vi "Main.vi"() -> ()   [LabVIEW 2012]
uses:
  UIActionQueueElement.ctl
  UIAction.ctl
  MemoryGlobalAction.ctl
  ScanListGlobalAction.ctl
  TriggerConfigurationGlobalAction.ctl
  SlotConfigurationGlobalAction.ctl
  Setup.ctl
  SlotConfiguration.ctl
  BankConfiguration.ctl
  TriggerConfiguration.ctl
  TriggerArmConfiguration.ctl
  driver/Public/Controls/ArmSource.ctl
  TriggerScanConfiguration.ctl
  driver/Public/Controls/ScanSource.ctl
  TriggerChannelConfiguration.ctl
  driver/Public/Controls/TriggerSource.ctl
  HardwareActionQueueElement.ctl
  HardwareAction.ctl
  libs/LV-Utilities/LV-Utilities.lvlib
  driver/Keithley-7001.lvlib
panel:
  in  "Tab Control":enum32{"Page 1"}(tab)
  out "Setup File":path
  in  "CONFIGURE SLOT 1":bool
  in  "CONFIGURE MEMORY":bool
  in  "CONFIGURE SCAN":bool
  in  "CONFIGURE TRIGGER":bool
  in  "Hardware START":bool
  out "Hardware Running?":bool
  in  "RESET":bool
  in  "SAVE":bool
  in  "OPEN":bool
  in  "DONE":bool
  # "RUN"
  # "SETUP"
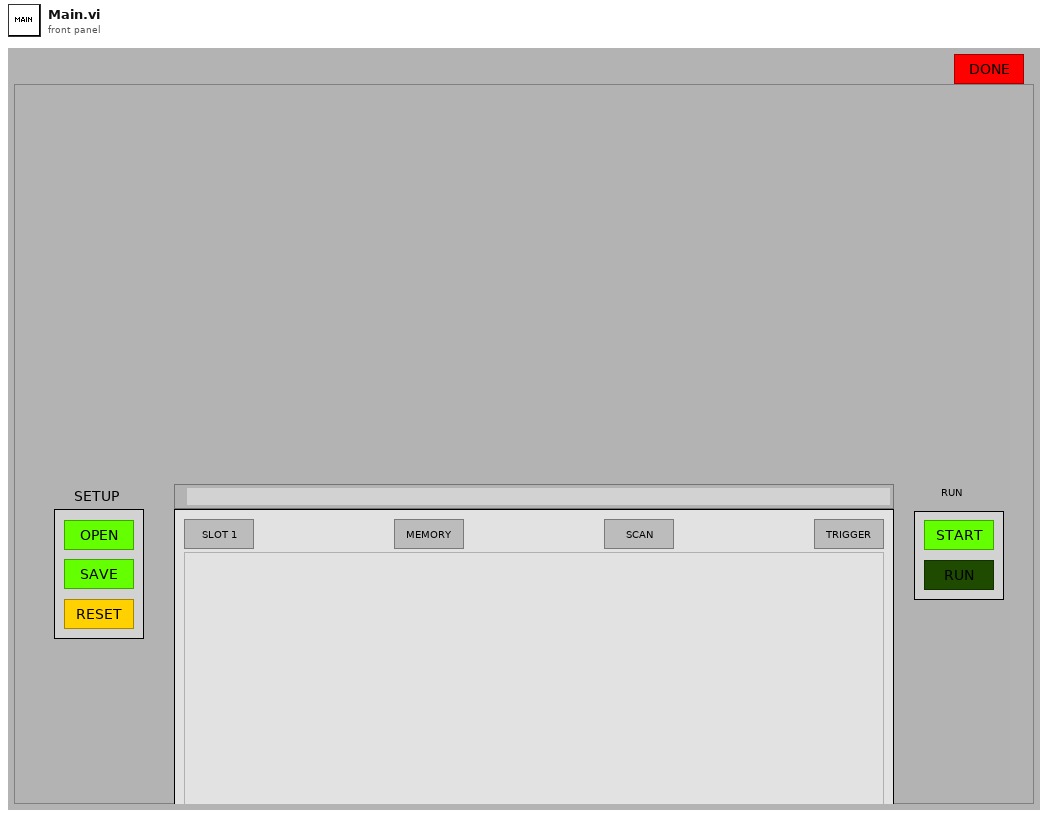
[diagram p1: front panel]
types:
  T1 = typedef "ActionQueues.ctl" = cluster{"User Interface":refnum<queue>, "Hardware":refnum<queue>}
  T2 = typedef "ExecutableConfiguration.ctl" = cluster{"GPIB ID":u8, "GPIB Board":u8, "Default Setup Folder":path}
  T3 = typedef "SlotConfigurationGlobalAction.ctl" = enum16{"Get", "Set", "Reset"}
  T4 = typedef "TriggerConfigurationGlobalAction.ctl" = enum16{"Get", "Set", "Reset"}
  T5 = typedef "ScanListGlobalAction.ctl" = enum16{"Get", "Set", "Reset"}
  T6 = typedef "MemoryGlobalAction.ctl" = enum16{"Get", "Set", "Reset"}
  T7 = typedef "Setup.ctl" = cluster{"Slots":T8[], "Memory":string[], "Scan List":string, "Trigger":T10}
  T8 = typedef "SlotConfiguration.ctl" = cluster{"Board":string, "Name":string, "Banks":T9[]}
  T9 = typedef "BankConfiguration.ctl" = cluster{"ID":string, "Name":string, "Channel Names":string[]}
  T10 = typedef "TriggerConfiguration.ctl" = cluster{"Arm":T11, "Scan":T13, "Channel":T15}
  T11 = typedef "TriggerArmConfiguration.ctl" = cluster{"Source":T12, "Count":u32, "Infinite?":bool}
  T12 = typedef "Keithley-7001.lvlib/ArmSource.ctl" = enum16{"Hold", "Immediate", "Manual", "Bus", "TLink", "External"}
  T13 = typedef "TriggerScanConfiguration.ctl" = cluster{"Source":T14, "Count":u32, "Infinite?":bool, "Delay (sec)":dbl, "Interval (sec)":dbl}
  T14 = typedef "Keithley-7001.lvlib/ScanSource.ctl" = enum16{"Hold", "Immediate", "Timer", "Manual", "Bus", "TLink", "External"}
  T15 = typedef "TriggerChannelConfiguration.ctl" = cluster{"Source":T16, "Count":u32, "Infinite?":bool, "Auto Count?":bool, "Delay (sec)":dbl, "Interval (sec)":dbl}
  T16 = typedef "Keithley-7001.lvlib/TriggerSource.ctl" = enum16{"Hold", "Immediate", "Manual", "Bus", "TLink", "External", "Timer"}
  T17 = typedef "HardwareActionQueueElement.ctl" = cluster{"Action":T18, "Data":variant}
  T18 = typedef "HardwareAction.ctl" = enum16{"Initialize", "Start", "Stop", "Error", "Shutdown"}
  T19 = typedef "UIActionQueueElement.ctl" = cluster{"Action":T20, "Data":variant}
  T20 = typedef "UIAction.ctl" = enum16{"Initialize", "Configure Trigger", "Configure Scan", "Configure Memory", "Configure Slot 1", "Open", "Save", "Reset", "Start", "Started", "Stop", "Stopped", "Shutdown"}
  T21 = enum8{"Enabled", "Disabled", "Disabled and Grayed Out"}
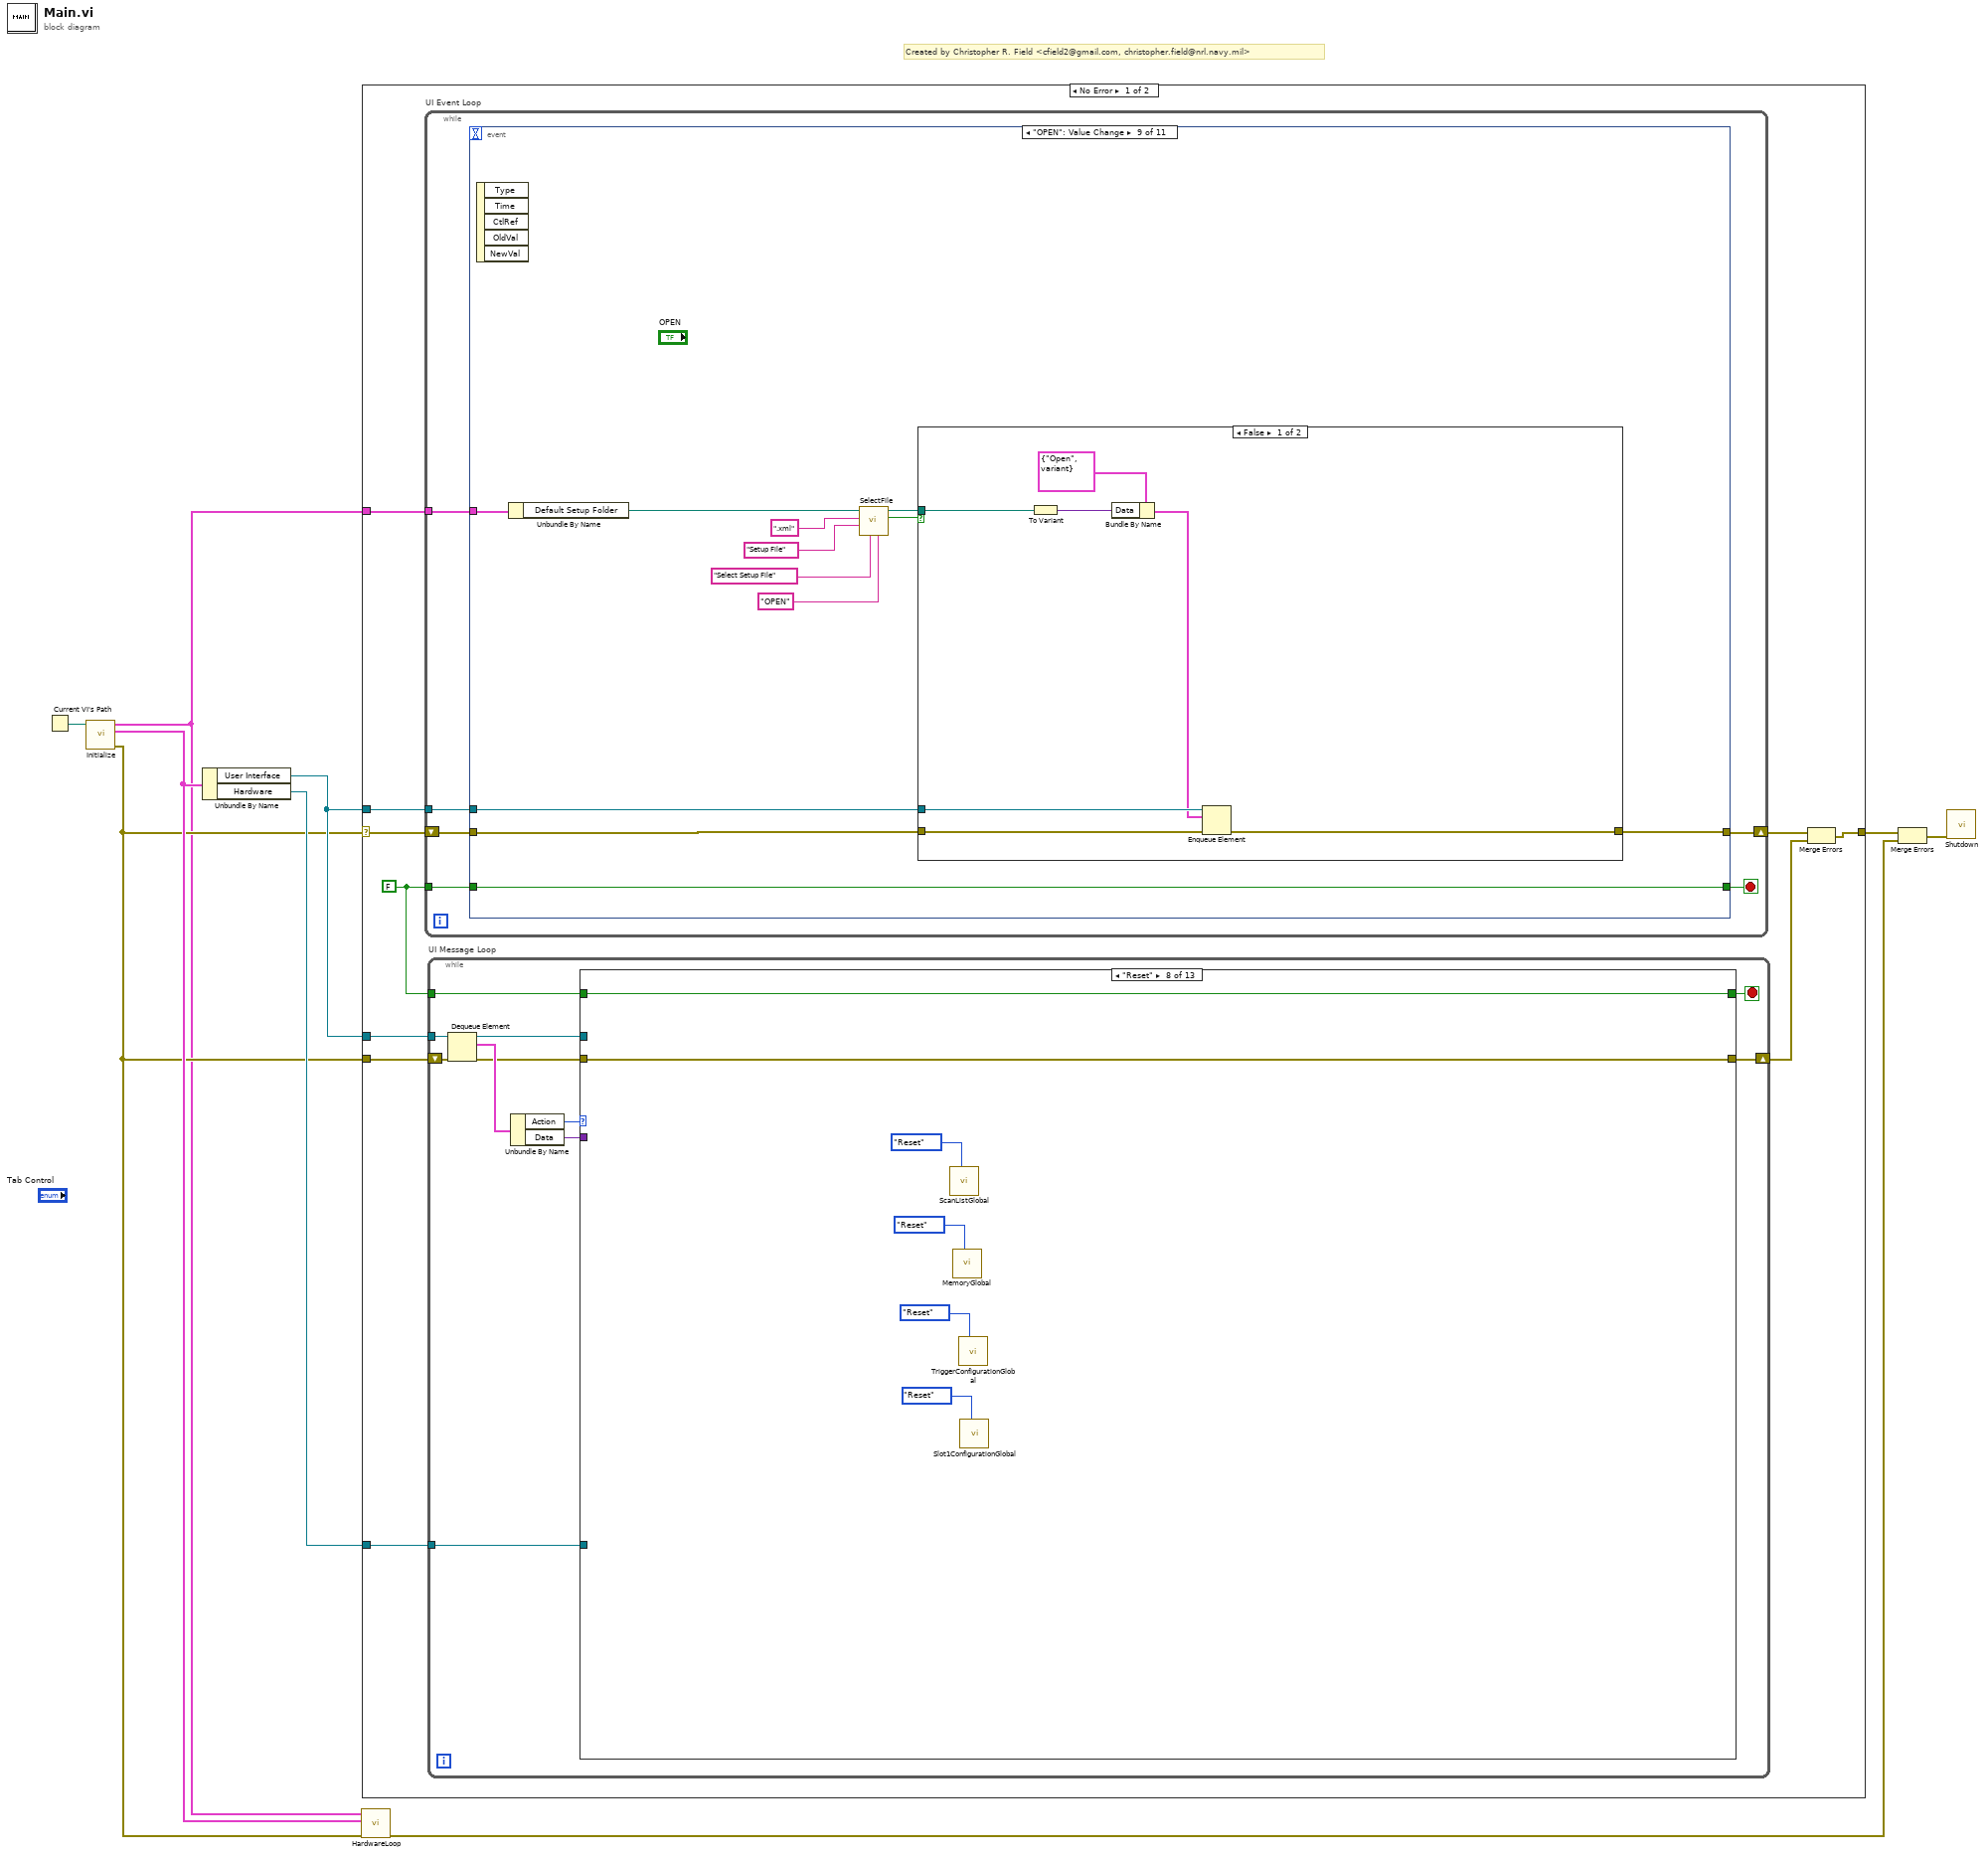
[diagram p0: block diagram]
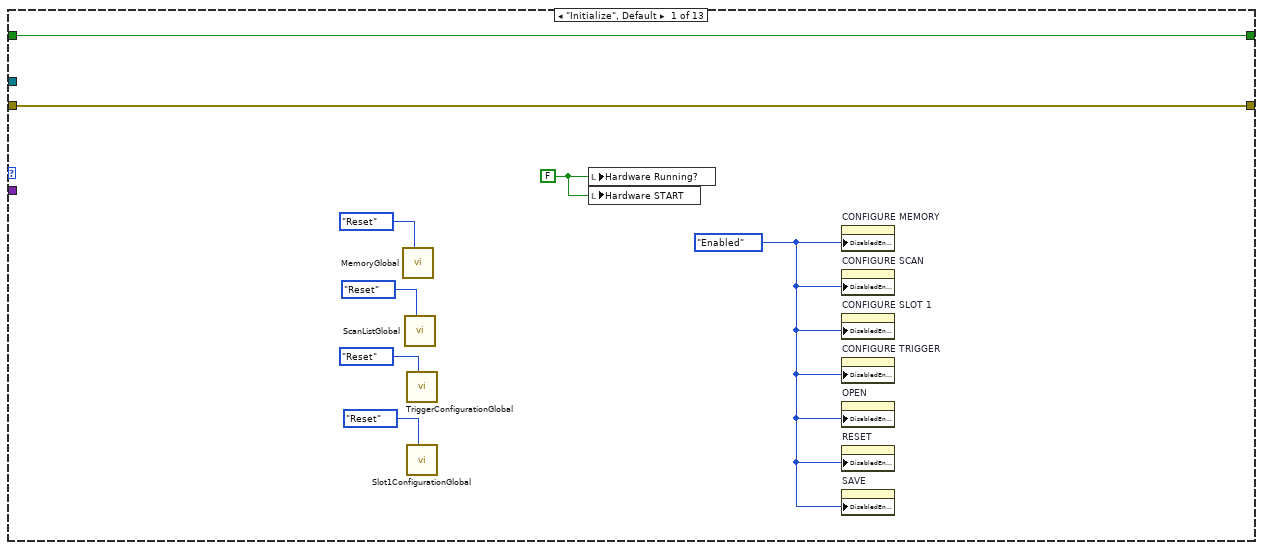
[diagram p2: hidden frame]
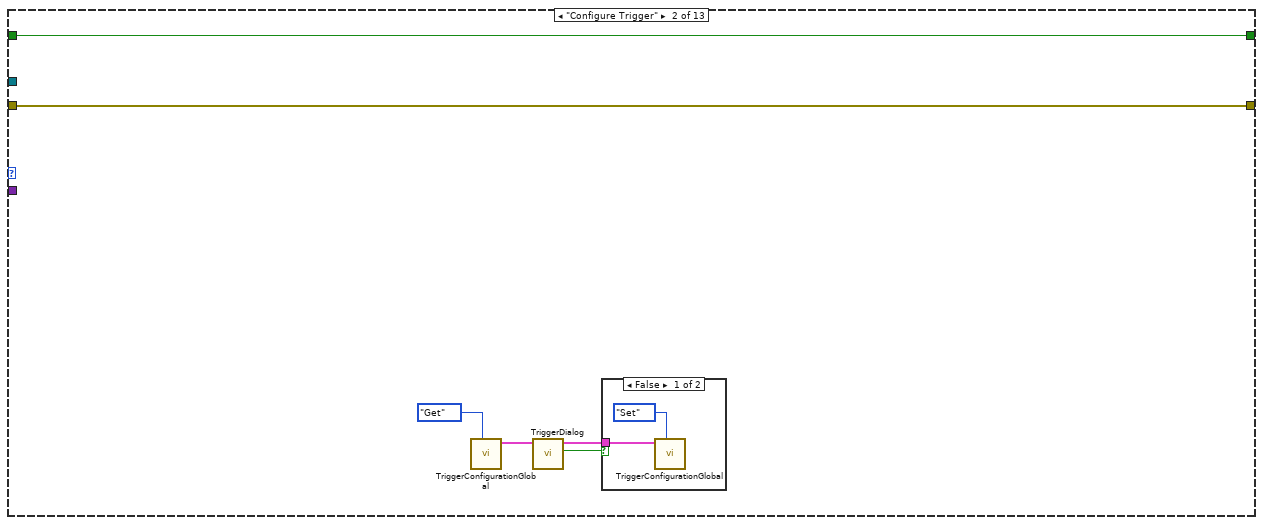
[diagram p3: hidden frame]
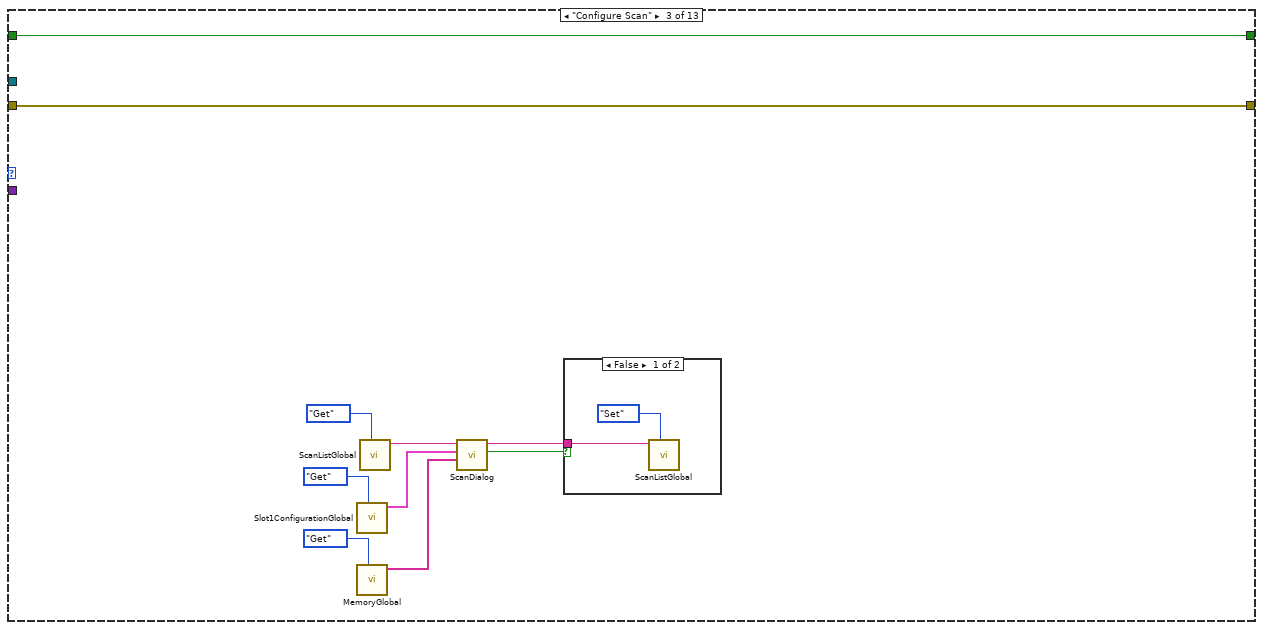
[diagram p5: hidden frame]
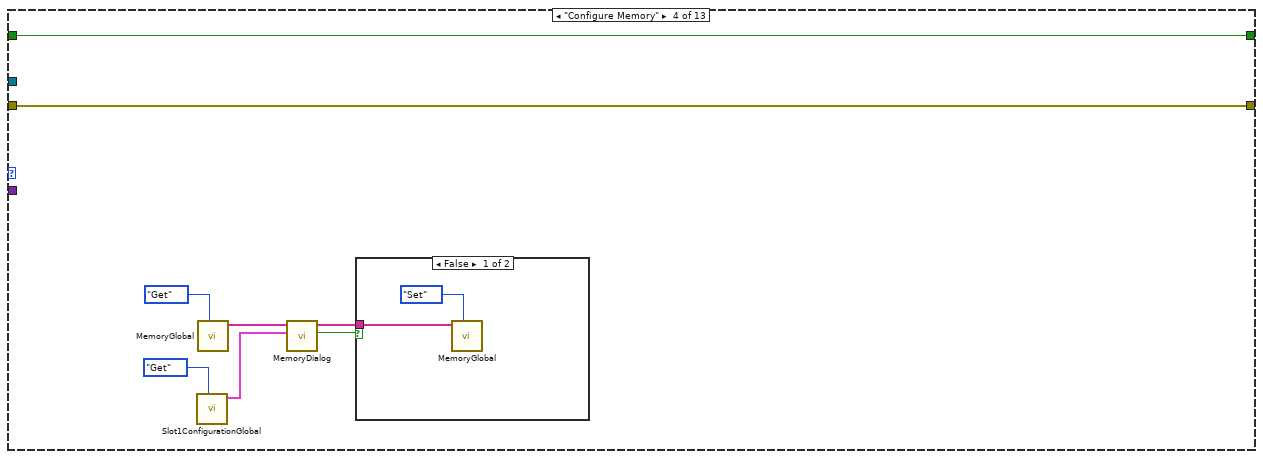
[diagram p7: hidden frame]
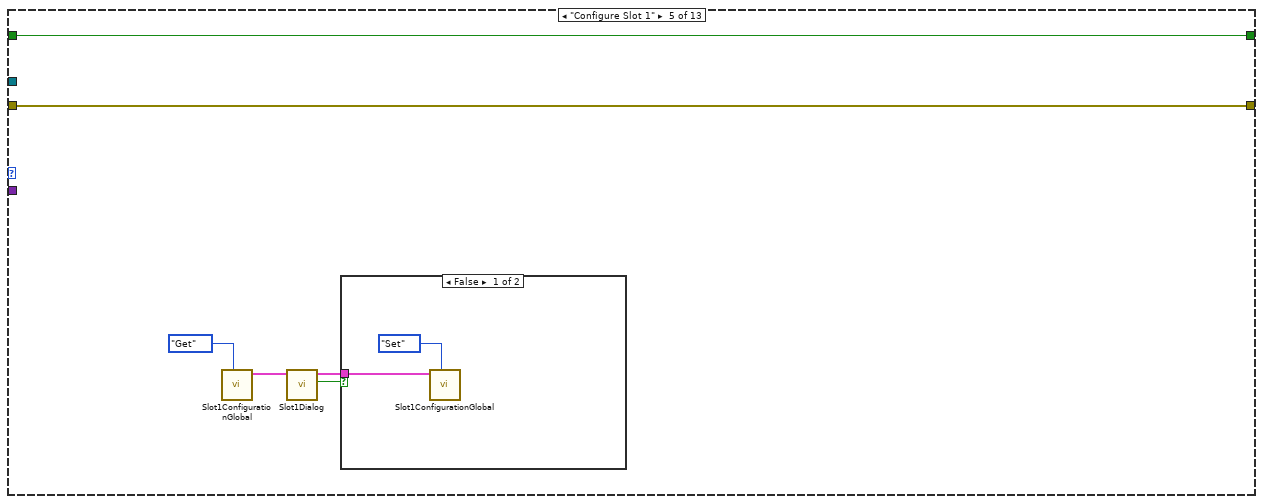
[diagram p9: hidden frame]
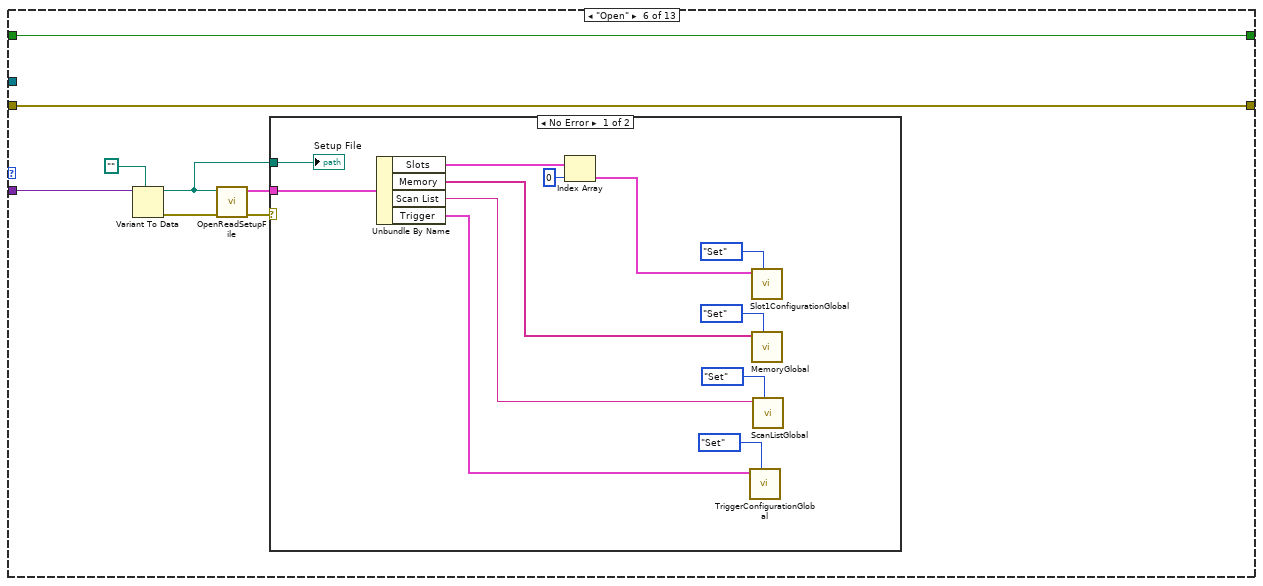
[diagram p11: hidden frame]
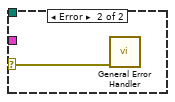
[diagram p12: hidden frame]
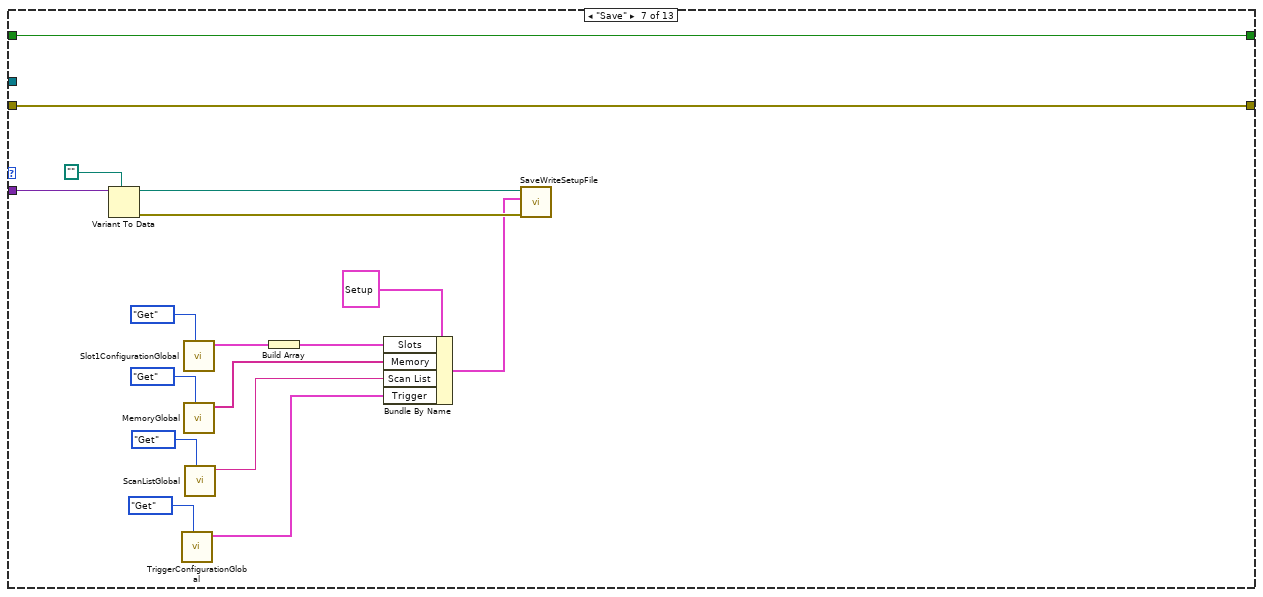
[diagram p13: hidden frame]
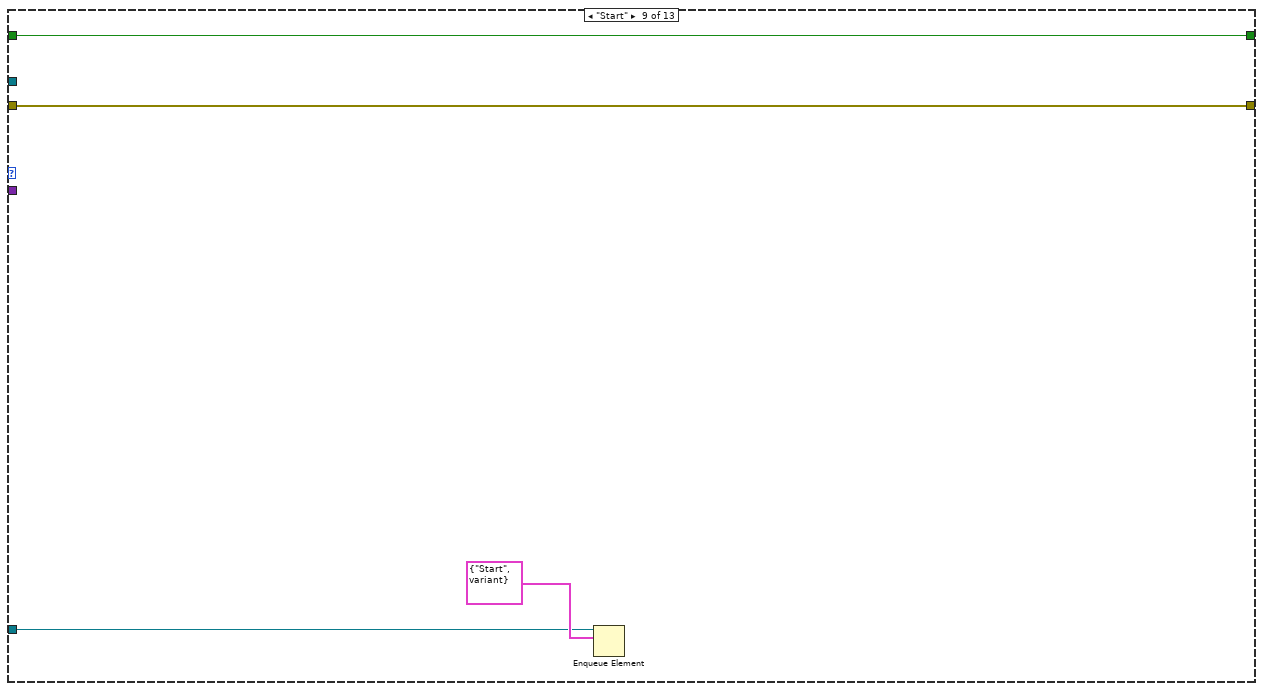
[diagram p14: hidden frame]
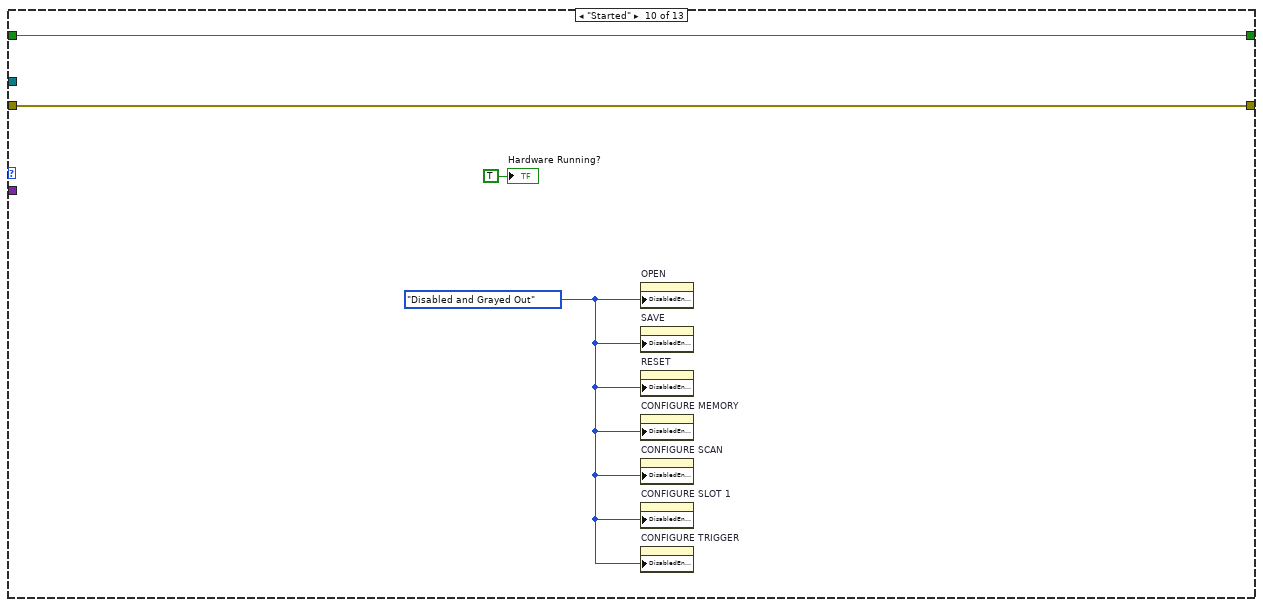
[diagram p15: hidden frame]
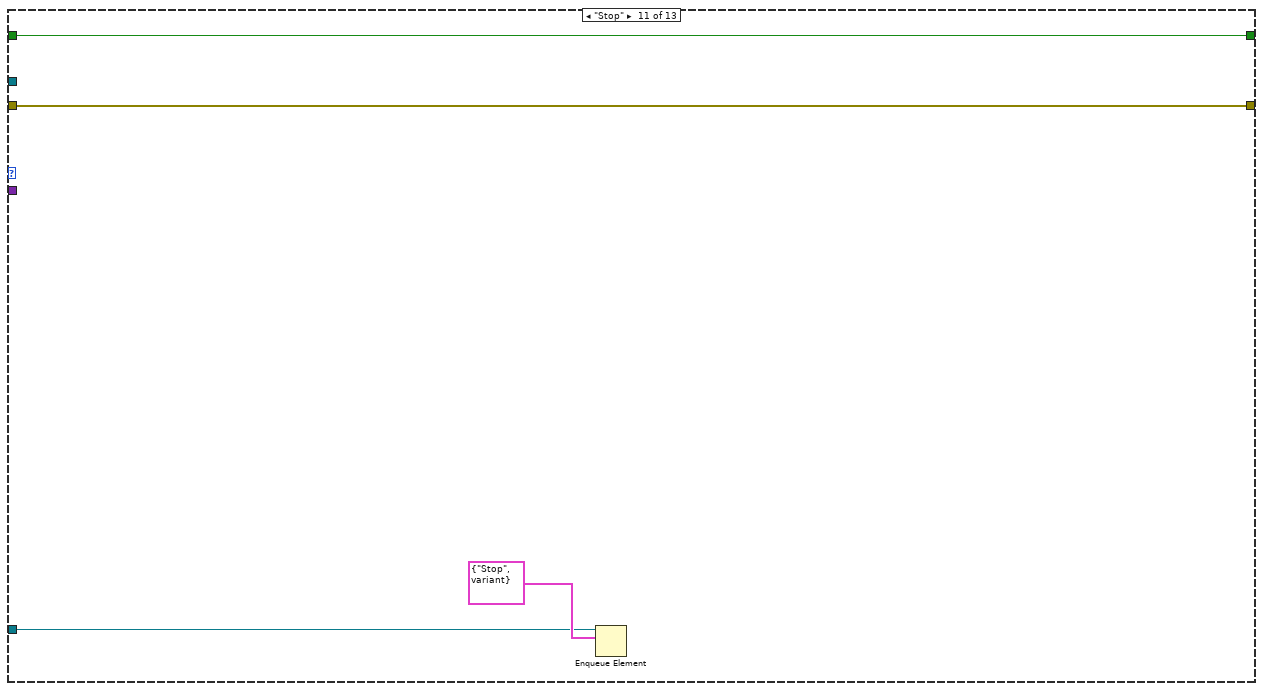
[diagram p16: hidden frame]
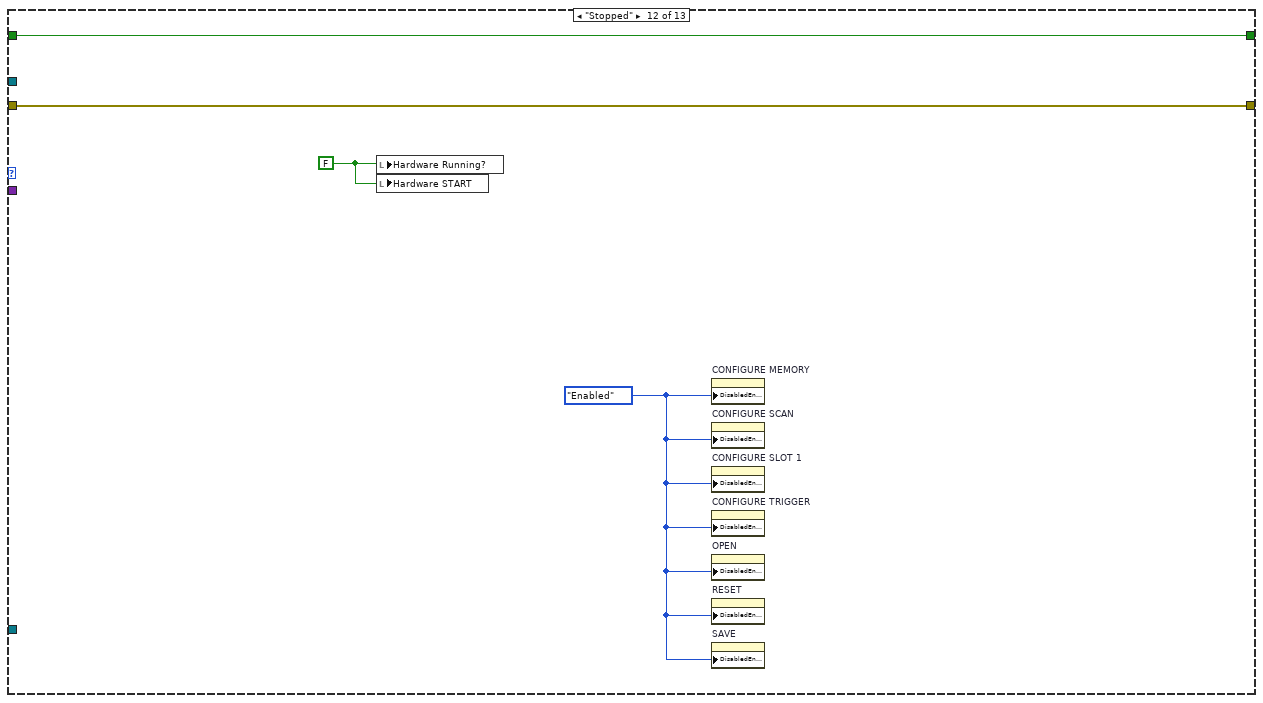
[diagram p17: hidden frame]
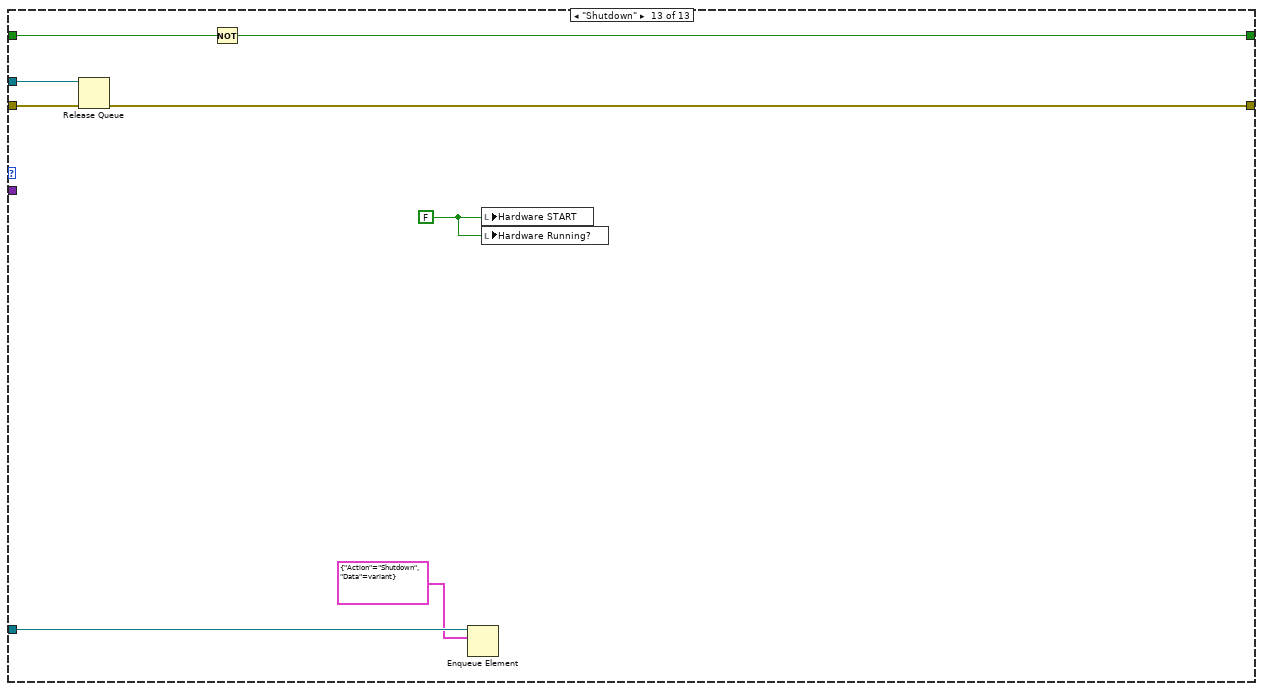
[diagram p18: hidden frame]
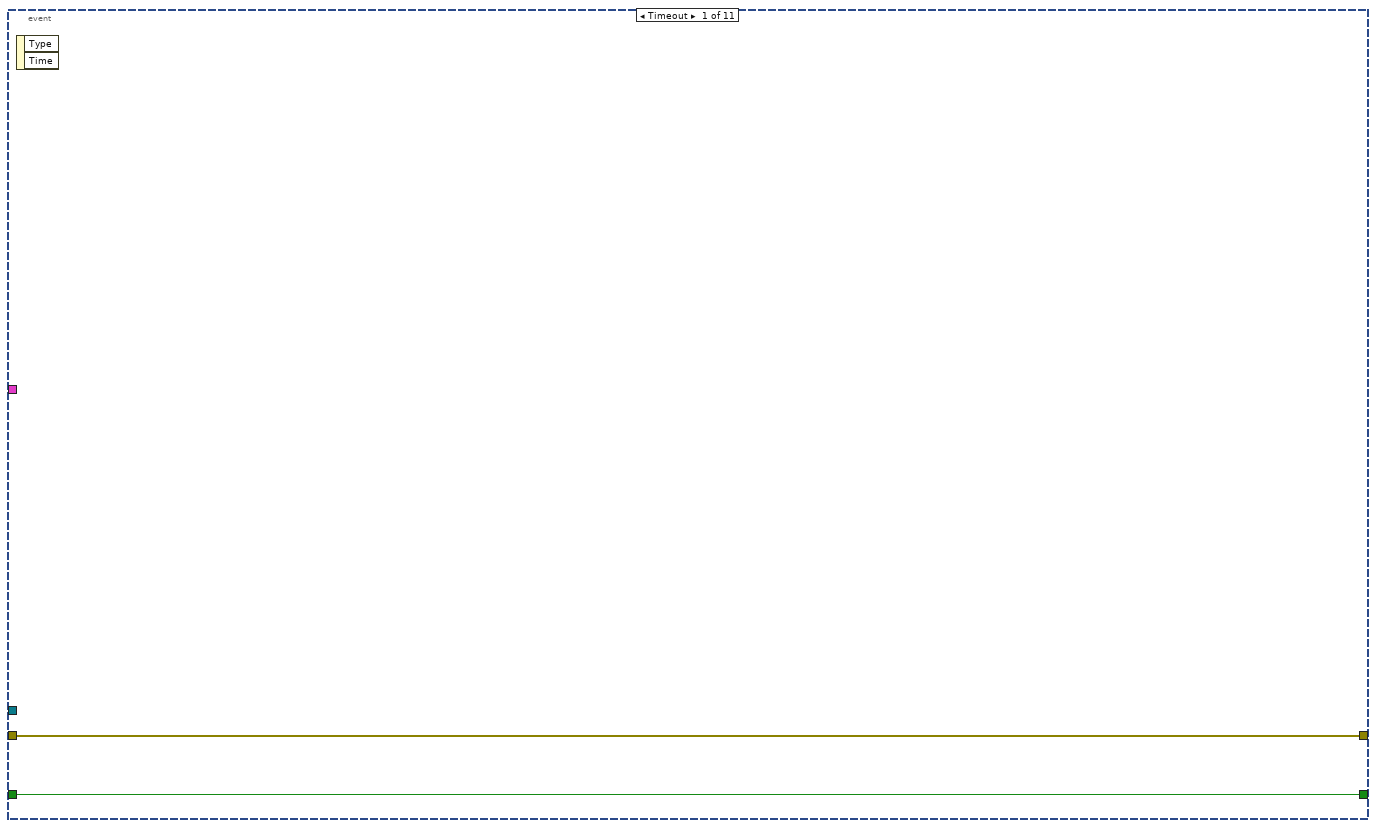
[diagram p19: hidden frame]
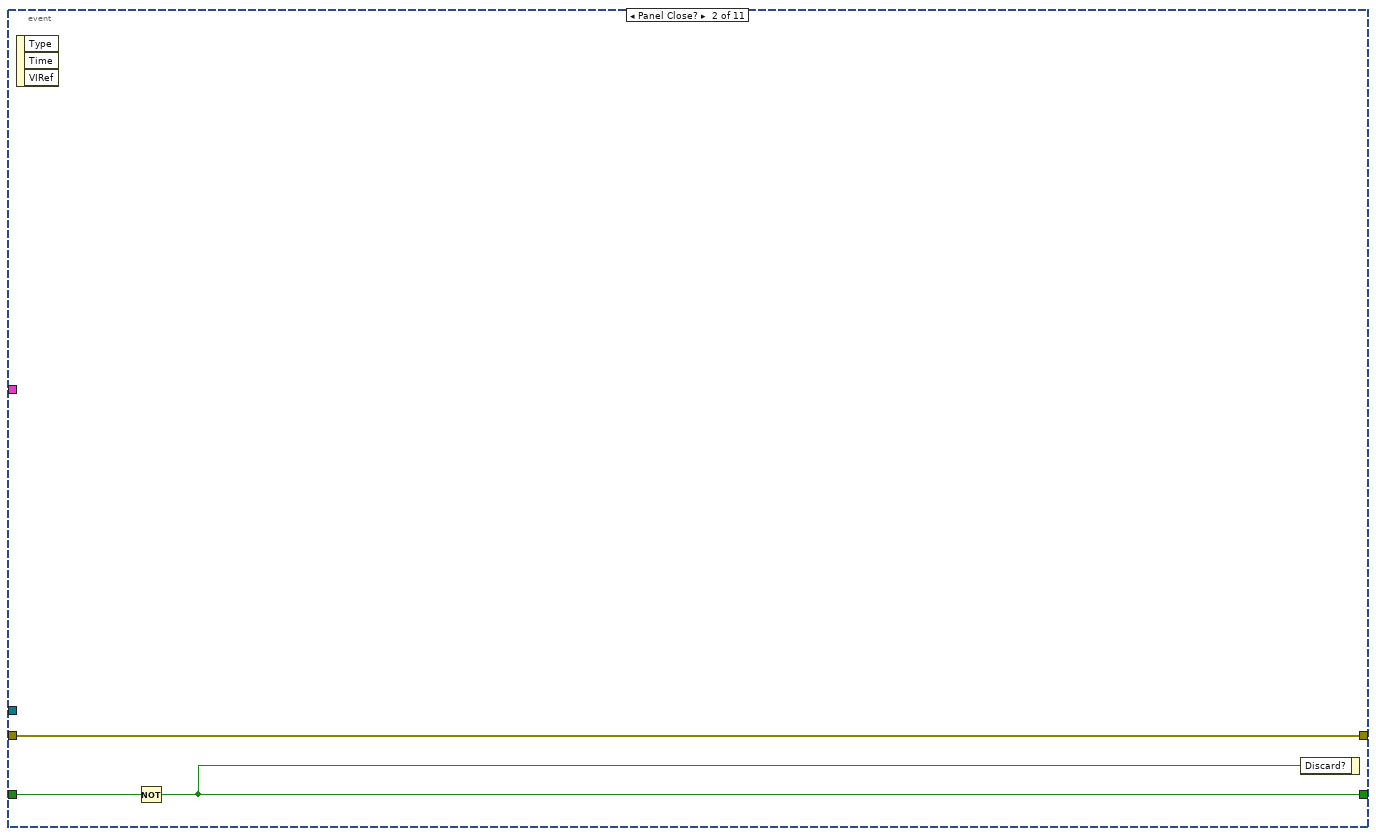
[diagram p20: hidden frame]
diagram:
  # "Created by Christopher R. Field <cfield2@gmail.com, christopher.field@nrl.navy.mil>"
  n1 = Current VI's Path() -> (path=w9:path)
  n2 = call "Initialize.vi"("VI Path"=w9) -> ("Error Out"=w5:errorcluster, "Action Queues"=w6:T1, "Executable Configuration"=w1:T2)  [unwired: 8 in]
  n3 = Unbundle By Name(w6) -> ("User Interface"=w8:refnum<queue>, "Hardware"=w7:refnum<queue>)
  n4 = call "HardwareLoop.vi"("Error In"=w5, "Action Queues"=w6, "Executable Configuration"=w1) -> ("Error Out"=w2:errorcluster)  [unwired: 8 in]
  n5 = case shown="No Error" w5 {
    selector: w5 -> [w19 w235]
    tunnel: [w12 w235] -> w4
    tunnel: w8 -> [w17 _]
    tunnel: w8 -> [w16 _]
    tunnel: w5 -> [w15 _]
    tunnel: w7 -> [w11 _]
    tunnel: w1 -> [w10 _]
    frame No Error {
      w18 = FALSE
      n6 = while "UI Event Loop" {
        shift-right: [w149] -> w14
        shift-left: w19 -> [w150]
        tunnel: w18 -> [w148]
        tunnel: w17 -> [w146]
        tunnel: w10 -> [w145]
        stop <- w147 stop-if-true
        n7 = event shown="[8] \"OPEN\": Value Change" {
          selector: _ -> [_ _ _ _ _ _ _ _ _ _ _]
          dyn-events: _ -> [_ _ _ _ _ _ _ _ _ _ _]
          timeout: _ -> [_ _ _ _ _ _ _ _ _ _ _]
          tunnel: w150 -> [w152 w155 w158 w165 w172 w178 w183 w187 w190 w212 w233]
          tunnel: [w152 w155 w157 w164 w168 w176 w182 w186 w191 w211 w232] -> w149
          tunnel: w148 -> [w151 w154 w161 w163 w167 w175 w181 w189 w195 w210 w231]
          tunnel: [w151 w153 w160 w163 w167 w175 w181 w189 w195 w210 w231] -> w147
          tunnel: w146 -> [_ _ w159 w166 w173 w179 w184 w188 w192 w213 w234]
          tunnel: w145 -> [_ _ _ _ _ _ _ _ w201 w214 _]
          event Timeout {
            n8 = event-data() -> ()  [unwired: 1 in, 2 out]
          }
          event Panel Close? {
            n9 = event-data() -> ()  [unwired: 1 in, 3 out]
            n10 = Not(x=w154) -> (.not. x?=w153:bool)
            n11 = event-data("Discard?"=w153) -> ()  [unwired: 1 in, 1 out]
          }
          event "DONE": Value Change {
            n12 = event-data() -> ()  [unwired: 1 in, 5 out]
            n13 = Not(x=w161) -> (.not. x?=w160:bool)
            n14 = Enqueue Element(queue=w159, element=T19 {"Action"=enum."Shutdown", "Data"=variant}, error in (no error)=w158) -> (error out=w157:errorcluster)  [unwired: 1 in, 2 out]
          }
          event "CONFIGURE TRIGGER": Value Change {
            n15 = event-data() -> ()  [unwired: 1 in, 5 out]
            n16 = Enqueue Element(queue=w166, element=T19 {"Action"=enum."Configure Trigger", "Data"=variant}, error in (no error)=w165) -> (error out=w164:errorcluster)  [unwired: 1 in, 2 out]
          }
          event "Hardware START": Value Change {
            n17 = event-data() -> ()  [unwired: 1 in, 5 out]
            n18 = Select(t=T19 {"Action"=enum."Start", "Data"=variant} ("element"), s="Hardware START", f=T19 {"Action"=enum."Stop", "Data"=variant} ("element")) -> (s? t:f=w169:T19)
            n19 = Enqueue Element(queue=w173, element=w169, error in (no error)=w172) -> (error out=w168:errorcluster)  [unwired: 1 in, 2 out]
          }
          event "CONFIGURE SCAN": Value Change {
            n20 = event-data() -> ()  [unwired: 1 in, 5 out]
            n21 = Enqueue Element(queue=w179, element=T19 {"Action"=enum."Configure Scan", "Data"=variant}, error in (no error)=w178) -> (error out=w176:errorcluster)  [unwired: 1 in, 2 out]
          }
          event "CONFIGURE MEMORY": Value Change {
            n22 = event-data() -> ()  [unwired: 1 in, 5 out]
            n23 = Enqueue Element(queue=w184, element=T19 {"Action"=enum."Configure Memory", "Data"=variant}, error in (no error)=w183) -> (error out=w182:errorcluster)  [unwired: 1 in, 2 out]
          }
          event "CONFIGURE SLOT 1": Value Change {
            n24 = event-data() -> ()  [unwired: 1 in, 5 out]
            n25 = Enqueue Element(queue=w188, element=T19 {"Action"=enum."Configure Slot 1", "Data"=variant}, error in (no error)=w187) -> (error out=w186:errorcluster)  [unwired: 1 in, 2 out]
          }
          event "OPEN": Value Change {
            n26 = event-data() -> ()  [unwired: 1 in, 5 out]
            n27 = Unbundle By Name(w201) -> ("Default Setup Folder"=w200:path)
            n28 = call "SelectFile.vi"("Button Label"="OPEN", "Prompt"="Select Setup File", "File Description"="Setup File", "File Extension (.*)"=".xml", "Start Path"=w200) -> ("Cancelled?"=w194:bool, "Selected File Path"=w193:path)  [unwired: 4 in, 1 out]
            n29 = case shown="False" w194 {
              tunnel: w193 -> [w203 _]
              tunnel: w192 -> [w208 _]
              tunnel: [w207 w209] -> w191
              tunnel: w190 -> [w206 w209]
              frame False {
                n30 = To Variant(anything=w203) -> (Variant=w204:variant)
                n31 = Bundle By Name(cluster=T19 {"Action"=enum."Open", "Data"=variant} ("element"), "Data"=w204) -> (w202:T19)
                n32 = Enqueue Element(queue=w208, element=w202, error in (no error)=w206) -> (error out=w207:errorcluster)  [unwired: 1 in, 2 out]
              }
              frame True {
              }
            }
          }
          event "SAVE": Value Change {
            n33 = event-data() -> ()  [unwired: 1 in, 5 out]
            n34 = Unbundle By Name(w214) -> ("Default Setup Folder"=w221:path)
            n35 = call "SelectFile.vi"("Button Label"="SAVE", "Prompt"="Select Setup File", "File Description"="Setup File", "File Extension (.*)"=".xml", "Start Path"=w221) -> ("Cancelled?"=w216:bool, "Selected File Path"=w215:path)  [unwired: 4 in, 1 out]
            n36 = case shown="False" w216 {
              tunnel: w215 -> [w223 _]
              tunnel: w213 -> [w228 _]
              tunnel: [w227 w229] -> w211
              tunnel: w212 -> [w226 w229]
              frame False {
                n37 = To Variant(anything=w223) -> (Variant=w224:variant)
                n38 = Bundle By Name(cluster=T19 {"Action"=enum."Save", "Data"=variant} ("element"), "Data"=w224) -> (w222:T19)
                n39 = Enqueue Element(queue=w228, element=w222, error in (no error)=w226) -> (error out=w227:errorcluster)  [unwired: 1 in, 2 out]
              }
              frame True {
              }
            }
          }
          event "RESET": Value Change {
            n40 = event-data() -> ()  [unwired: 1 in, 5 out]
            n41 = Enqueue Element(queue=w234, element=T19 {"Action"=enum."Reset", "Data"=variant}, error in (no error)=w233) -> (error out=w232:errorcluster)  [unwired: 1 in, 2 out]
          }
        }
      }
      n42 = while "UI Message Loop" {
        tunnel: w18 -> [w30]
        tunnel: w16 -> [w29]
        shift-right: [w22] -> w13
        shift-left: w15 -> [w28]
        tunnel: w11 -> [w20]
        stop <- w21 stop-if-true
        n43 = Dequeue Element(queue=w29, error in (no error)=w28) -> (queue out=w23:refnum<queue>, element=w27:T19, error out=w24:errorcluster)  [unwired: 1 in, 1 out]
        n44 = Unbundle By Name(w27) -> ("Action"=w26:T20, "Data"=w25:variant)
        n45 = case shown="\"Reset\"" w26 {
          tunnel: w30 -> [w38 w43 w56 w66 w73 w84 w113 w120 w124 w128 w132 w136 w144]
          tunnel: w25 -> [_ _ _ _ _ w82 w112 _ _ _ _ _ _]
          tunnel: w24 -> [w37 w44 w55 w65 w74 w83 w114 w119 w123 w127 w131 w135 w141]
          tunnel: w23 -> [_ _ _ _ _ _ _ _ _ _ _ _ w142]
          tunnel: [w37 w44 w55 w65 w74 w83 w114 w119 w123 w127 w131 w135 w140] -> w22
          tunnel: [w38 w43 w56 w66 w73 w84 w113 w120 w124 w128 w132 w136 w143] -> w21
          tunnel: w20 -> [_ _ _ _ _ _ _ _ w121 _ w129 _ w139]
          frame "Initialize", Default {
            w31 = T21."Enabled" ("Disabled")
            w36 = FALSE ("Hardware Running?")
            n46 = call "MemoryGlobal.vi"("Action"=MemoryGlobalAction."Reset") -> ()  [unwired: 10 in, 1 out]
            n47 = call "ScanListGlobal.vi"("Action"=ScanListGlobalAction."Reset") -> ()  [unwired: 10 in, 1 out]
            n48 = call "TriggerConfigurationGlobal.vi"("Action"=TriggerConfigurationGlobalAction."Reset") -> ()  [unwired: 10 in, 1 out]
            n49 = call "Slot1ConfigurationGlobal.vi"("Action"=SlotConfigurationGlobalAction."Reset") -> ()  [unwired: 10 in, 1 out]
            n50 = local write "Hardware Running?"(w36) -> ()
            n51 = local write "Hardware START"(w36) -> ()
            n52 = property on="CONFIGURE MEMORY" class="Bool"("DisabledEnum"=w31) -> ()  [unwired: 2 in, 2 out]
            n53 = property on="CONFIGURE SCAN" class="Bool"("DisabledEnum"=w31) -> ()  [unwired: 2 in, 2 out]
            n54 = property on="CONFIGURE SLOT 1" class="Bool"("DisabledEnum"=w31) -> ()  [unwired: 2 in, 2 out]
            n55 = property on="CONFIGURE TRIGGER" class="Bool"("DisabledEnum"=w31) -> ()  [unwired: 2 in, 2 out]
            n56 = property on="OPEN" class="Bool"("DisabledEnum"=w31) -> ()  [unwired: 2 in, 2 out]
            n57 = property on="RESET" class="Bool"("DisabledEnum"=w31) -> ()  [unwired: 2 in, 2 out]
            n58 = property on="SAVE" class="Bool"("DisabledEnum"=w31) -> ()  [unwired: 2 in, 2 out]
          }
          frame "Configure Trigger" {
            n59 = call "TriggerConfigurationGlobal.vi"("Action"=TriggerConfigurationGlobalAction."Get") -> ("Value Out"=w41:T10)  [unwired: 10 in]
            n60 = call "TriggerDialog.vi"("Trigger Configuration In"=w41) -> ("Cancelled?"=w39:bool, "Trigger Configuration Out"=w40:T10)  [unwired: 8 in, 1 out]
            n61 = case shown="False" w39 {
              tunnel: w40 -> [w46 _]
              frame False {
                n62 = call "TriggerConfigurationGlobal.vi"("Action"=TriggerConfigurationGlobalAction."Set", "Set Value"=w46) -> ()  [unwired: 9 in, 1 out]
              }
              frame True {
              }
            }
          }
          frame "Configure Scan" {
            n63 = call "Slot1ConfigurationGlobal.vi"("Action"=SlotConfigurationGlobalAction."Get") -> ("Value Out"=w49:T8)  [unwired: 10 in]
            n64 = call "MemoryGlobal.vi"("Action"=MemoryGlobalAction."Get") -> ("Value Out"=w47:string[])  [unwired: 10 in]
            n65 = call "ScanListGlobal.vi"("Action"=ScanListGlobalAction."Get") -> ("Value Out"=w53:string)  [unwired: 10 in]
            n66 = call "ScanDialog.vi"("Channel Patterns"=w47, "Slot Configuration"=w49, "Scan List In"=w53) -> ("Cancelled?"=w51:bool, "Scan List Out"=w52:string)  [unwired: 6 in, 1 out]
            n67 = case shown="False" w51 {
              tunnel: w52 -> [w57 _]
              frame False {
                n68 = call "ScanListGlobal.vi"("Action"=ScanListGlobalAction."Set", "Set Value"=w57) -> ()  [unwired: 9 in, 1 out]
              }
              frame True {
              }
            }
          }
          frame "Configure Memory" {
            n69 = call "Slot1ConfigurationGlobal.vi"("Action"=SlotConfigurationGlobalAction."Get") -> ("Value Out"=w59:T8)  [unwired: 10 in]
            n70 = call "MemoryGlobal.vi"("Action"=MemoryGlobalAction."Get") -> ("Value Out"=w63:string[])  [unwired: 10 in]
            n71 = call "MemoryDialog.vi"("Slot 1 Configuration"=w59, "Channel Patterns In"=w63) -> ("Cancelled?"=w62:bool, "Channel Patterns Out"=w61:string[])  [unwired: 7 in, 1 out]
            n72 = case shown="False" w62 {
              tunnel: w61 -> [w68 _]
              frame False {
                n73 = call "MemoryGlobal.vi"("Action"=MemoryGlobalAction."Set", "Set Value"=w68) -> ()  [unwired: 9 in, 1 out]
              }
              frame True {
              }
            }
          }
          frame "Configure Slot 1" {
            n74 = call "Slot1ConfigurationGlobal.vi"("Action"=SlotConfigurationGlobalAction."Get") -> ("Value Out"=w71:T8)  [unwired: 10 in]
            n75 = call "Slot1Dialog.vi"("Slot 1 Configuration In"=w71) -> ("Cancelled?"=w70:bool, "Slot 1 Configuration Out"=w69:T8)  [unwired: 8 in, 1 out]
            n76 = case shown="False" w70 {
              tunnel: w69 -> [w76 _]
              frame False {
                n77 = call "Slot1ConfigurationGlobal.vi"("Action"=SlotConfigurationGlobalAction."Set", "Set Value"=w76) -> ()  [unwired: 9 in, 1 out]
              }
              frame True {
              }
            }
          }
          frame "Open" {
            n78 = Variant To Data(type=path "", Variant=w82) -> (data=w79:path, error out=w80:errorcluster)  [unwired: 1 in]
            n79 = call "OpenReadSetupFile.vi"("Error In"=w80, "Setup File"=w79) -> ("Error Out"=w78:errorcluster, "Setup"=w77:T7)  [unwired: 8 in]
            n80 = case shown="No Error" w78 {
              selector: w78 -> [_ w97]
              tunnel: w79 -> [w96 _]
              tunnel: w77 -> [w95 _]
              frame No Error {
                n81 = Unbundle By Name(w95) -> ("Slots"=w90:T8[], "Memory"=w87:string[], "Scan List"=w86:string, "Trigger"=w85:T10)
                n82 = Index Array(array=w90, index=0) -> (element=w88:T8)
                n83 = call "TriggerConfigurationGlobal.vi"("Action"=TriggerConfigurationGlobalAction."Set", "Set Value"=w85) -> ()  [unwired: 9 in, 1 out]
                n84 = call "Slot1ConfigurationGlobal.vi"("Action"=SlotConfigurationGlobalAction."Set", "Set Value"=w88) -> ()  [unwired: 9 in, 1 out]
                n85 = call "MemoryGlobal.vi"("Action"=MemoryGlobalAction."Set", "Set Value"=w87) -> ()  [unwired: 9 in, 1 out]
                n86 = call "ScanListGlobal.vi"("Action"=ScanListGlobalAction."Set", "Set Value"=w86) -> ()  [unwired: 9 in, 1 out]
                "Setup File" <- w96
              }
              frame Error {
                n87 = call <vilib>:"General Error Handler.vi"("error in (no error)"=w97) -> ()  [unwired: 10 in, 5 out]
              }
            }
          }
          frame "Save" {
            n88 = Variant To Data(type=path "", Variant=w112) -> (data=w110:path, error out=w109:errorcluster)  [unwired: 1 in]
            n89 = call "TriggerConfigurationGlobal.vi"("Action"=TriggerConfigurationGlobalAction."Get") -> ("Value Out"=w100:T10)  [unwired: 10 in]
            n90 = call "Slot1ConfigurationGlobal.vi"("Action"=SlotConfigurationGlobalAction."Get") -> ("Value Out"=w99:T8)  [unwired: 10 in]
            n91 = call "MemoryGlobal.vi"("Action"=MemoryGlobalAction."Get") -> ("Value Out"=w104:string[])  [unwired: 10 in]
            n92 = call "ScanListGlobal.vi"("Action"=ScanListGlobalAction."Get") -> ("Value Out"=w101:string)  [unwired: 10 in]
            n93 = Build Array(w99) -> (w98:T8[])
            n94 = Bundle By Name(cluster=T7 {"Slots"=[], "Memory"=[], "Scan List"="", "Trigger"={"Arm"={"Source"=enum."Hold", "Count"=0, "Infinite?"=FALSE}, "Scan"={"Source"=enum."Hold", "Count"=0, "Infinite?"=FALSE, "Delay (sec)"=0.0, "Interval (sec)"=0.0}, "Channel"={"Source"=enum."Hold", "Count"=0, "Infinite?"=FALSE, "Auto Count?"=FALSE, "Delay (sec)"=0.0, "Interval (sec)"=0.0}}} ("Setup"), "Slots"=w98, "Memory"=w104, "Scan List"=w101, "Trigger"=w100) -> (w106:T7)
            n95 = call "SaveWriteSetupFile.vi"("Error In"=w109, "Setup"=w106, "Save File"=w110) -> ()  [unwired: 8 in, 1 out]
          }
          frame "Reset" {
            n96 = call "ScanListGlobal.vi"("Action"=ScanListGlobalAction."Reset") -> ()  [unwired: 10 in, 1 out]
            n97 = call "MemoryGlobal.vi"("Action"=MemoryGlobalAction."Reset") -> ()  [unwired: 10 in, 1 out]
            n98 = call "TriggerConfigurationGlobal.vi"("Action"=TriggerConfigurationGlobalAction."Reset") -> ()  [unwired: 10 in, 1 out]
            n99 = call "Slot1ConfigurationGlobal.vi"("Action"=SlotConfigurationGlobalAction."Reset") -> ()  [unwired: 10 in, 1 out]
          }
          frame "Start" {
            n100 = Enqueue Element(queue=w121, element=T17 {"Action"=enum."Start", "Data"=variant}) -> ()  [unwired: 2 in, 3 out]
          }
          frame "Started" {
            w125 = T21."Disabled and Grayed Out" ("Disabled")
            n101 = property on="OPEN" class="Bool"("DisabledEnum"=w125) -> ()  [unwired: 2 in, 2 out]
            n102 = property on="SAVE" class="Bool"("DisabledEnum"=w125) -> ()  [unwired: 2 in, 2 out]
            n103 = property on="RESET" class="Bool"("DisabledEnum"=w125) -> ()  [unwired: 2 in, 2 out]
            n104 = property on="CONFIGURE MEMORY" class="Bool"("DisabledEnum"=w125) -> ()  [unwired: 2 in, 2 out]
            n105 = property on="CONFIGURE SCAN" class="Bool"("DisabledEnum"=w125) -> ()  [unwired: 2 in, 2 out]
            n106 = property on="CONFIGURE SLOT 1" class="Bool"("DisabledEnum"=w125) -> ()  [unwired: 2 in, 2 out]
            n107 = property on="CONFIGURE TRIGGER" class="Bool"("DisabledEnum"=w125) -> ()  [unwired: 2 in, 2 out]
            "Hardware Running?" <- TRUE ("Hardware Running?")
          }
          frame "Stop" {
            n108 = Enqueue Element(queue=w129, element=T17 {"Action"=enum."Stop", "Data"=variant}) -> ()  [unwired: 2 in, 3 out]
          }
          frame "Stopped" {
            w133 = T21."Enabled" ("Disabled")
            w134 = FALSE ("Hardware Running?")
            n109 = local write "Hardware Running?"(w134) -> ()
            n110 = local write "Hardware START"(w134) -> ()
            n111 = property on="CONFIGURE MEMORY" class="Bool"("DisabledEnum"=w133) -> ()  [unwired: 2 in, 2 out]
            n112 = property on="CONFIGURE SCAN" class="Bool"("DisabledEnum"=w133) -> ()  [unwired: 2 in, 2 out]
            n113 = property on="CONFIGURE SLOT 1" class="Bool"("DisabledEnum"=w133) -> ()  [unwired: 2 in, 2 out]
            n114 = property on="CONFIGURE TRIGGER" class="Bool"("DisabledEnum"=w133) -> ()  [unwired: 2 in, 2 out]
            n115 = property on="OPEN" class="Bool"("DisabledEnum"=w133) -> ()  [unwired: 2 in, 2 out]
            n116 = property on="RESET" class="Bool"("DisabledEnum"=w133) -> ()  [unwired: 2 in, 2 out]
            n117 = property on="SAVE" class="Bool"("DisabledEnum"=w133) -> ()  [unwired: 2 in, 2 out]
          }
          frame "Shutdown" {
            w137 = FALSE ("Hardware START")
            n118 = Release Queue(queue=w142, error in (no error)=w141) -> (error out=w140:errorcluster)  [unwired: 1 in, 2 out]
            n119 = Not(x=w144) -> (.not. x?=w143:bool)
            n120 = Enqueue Element(queue=w139, element=T17 {"Action"=enum."Shutdown", "Data"=variant}) -> ()  [unwired: 2 in, 3 out]
            n121 = local write "Hardware START"(w137) -> ()
            n122 = local write "Hardware Running?"(w137) -> ()
          }
        }
      }
      n123 = Merge Errors(w14, w13) -> (w12:errorcluster)
    }
    frame Error {
    }
  }
  n124 = Merge Errors(w4, w2) -> (w3:errorcluster)
  n125 = call "Shutdown.vi"("Error In"=w3) -> ()  [unwired: 10 in, 1 out]
